vi "Get Files and Folders.vi"(0 "File Directory":path, 11 "error in (no error)":errorcluster) -> (4 "Files and Folders":path[](array[path]), 6 "Files and Folder Names":string[](array[string]), 15 "error out":errorcluster)   [LabVIEW 2021, in "Packager Helpers.lvlib"]
uses:
  Packager Helpers.lvlib
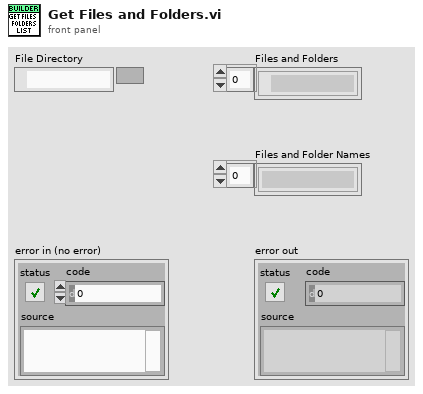
[diagram p1: front panel]
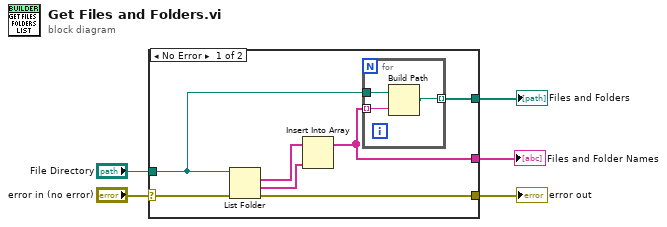
[diagram p0: block diagram]
diagram:
  n1 = case shown="No Error" "error in (no error)" {
    selector: "error in (no error)" -> [w6 w16]
    tunnel: [w12 _] -> w5
    tunnel: [w11 _] -> w4
    tunnel: "File Directory" -> [w10 _]
    tunnel: [w7 w16] -> w2
    frame No Error {
      n2 = List Folder(path=w10, error in=w6) -> (filenames=w9:string[], folder names=w8:string[], error out=w7:errorcluster)  [unwired: 2 in, 1 out]
      n3 = Insert Into Array(array=w9, new element=w8) -> (w11:string[])  [unwired: 1 in]
      n4 = for {
        tunnel: w10 -> [w15]
        tunnel: w11 -> [w14] mode=indexing
        tunnel: [w13] -> w12 mode=indexing
        n5 = Build Path(base path=w15, name or relative path=w14) -> (appended path=w13:path)
      }
    }
    frame Error {
    }
  }
  "Files and Folders" <- w5
  "error out" <- w2
  "Files and Folder Names" <- w4
